vi "Update Message Count.vi"(7 "I2C Messages Count Ref":refnum<vi>, 8 "error in (no error)":errorcluster, 11 "Fetch Count Ref":refnum<vi>) -> (0 "error out":errorcluster)   [LabVIEW 2025, in "I2C Bus Monitor UI.lvlib"]
uses:
  I2C Bus Monitor UI.lvlib
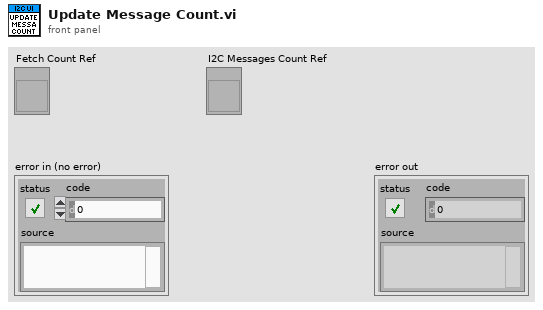
[diagram p1: front panel]
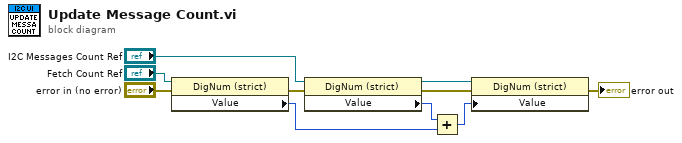
[diagram p0: block diagram]
diagram:
  n1 = property class="DigNum (strict)"(reference="Fetch Count Ref", error in="error in (no error)") -> (error out=w3:errorcluster, "Value"=w1:i32)  [unwired: 1 out]
  n2 = property on="Property Node" class="DigNum (strict)"(reference="I2C Messages Count Ref", error in=w3) -> (reference out=w5:refnum<vi>, error out=w4:errorcluster, "Value"=w6:i32)
  n3 = Add(x=w6, y=w1) -> (x+y=w7:i32)
  n4 = property on="Property Node" class="DigNum (strict)"(reference=w5, error in=w4, "Value"=w7) -> (error out=→"error out":errorcluster)  [unwired: 1 out]
